vi "Publish Update.vi"(8 "error in (no error)":errorcluster, 11 "DAQmxDO in":refnum<class "DAQmxDO.lvclass">) -> (0 "error out":errorcluster, 3 "DAQmxDO out":refnum<class "DAQmxDO.lvclass">)   [LabVIEW 2020, in "VolatusDAQ.lvlib" / "DAQmxDO.lvclass"]
uses:
  DAQmxDO.lvclass
  DAQmxDO.lvclass/DAQmxDO.ctl
  VolatusData/VolatusData.lvlib
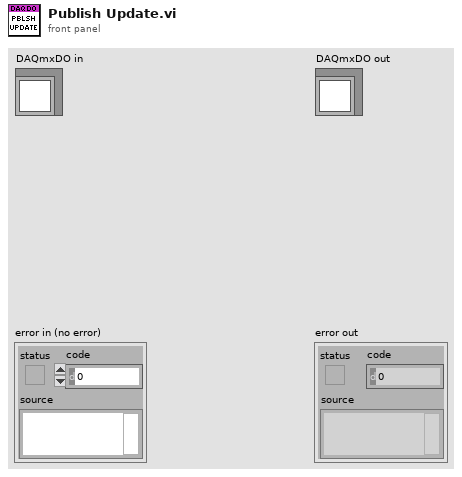
[diagram p1: front panel]
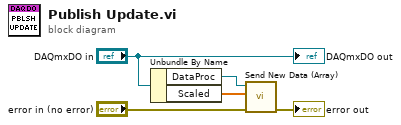
[diagram p0: block diagram]
diagram:
  n1 = Unbundle By Name("DAQmxDO in") -> ("DataProc"=w5:refnum<class "MessageQ.lvclass">, "Scaled"=w4:dbl[])
  n2 = call "Send New Data (Array).vi"("error in (no error)"="error in (no error)", "Data"=w4, "MessageQ"=w5) -> ("error out"=→"error out":errorcluster)  [unwired: 8 in]
  "DAQmxDO out" <- "DAQmxDO in"
